vi "Grab Image.vi"(8 "error in (no error)":errorcluster, 11 "Bobcat 640 in":refnum<class "Bobcat 640.lvclass">) -> (0 "error out":errorcluster, 3 "Bobcat 640 out":refnum<class "Bobcat 640.lvclass">)   [LabVIEW 2018, in "Bobcat 640.lvlib" / "Bobcat 640.lvclass"]
uses:
  Bobcat 640.lvclass
  Bobcat 640.lvclass/Bobcat 640.ctl
  PPLs/Camera/Parent/Camera.lvlibp/Camera.lvclass
  <vilib>/vision/driver/NI_Vision_Acquisition_Software.lvlib
  C:/AME Test Engineering/LabVIEW/PPLs/Camera/Parent/Camera.lvlibp/Camera.lvclass
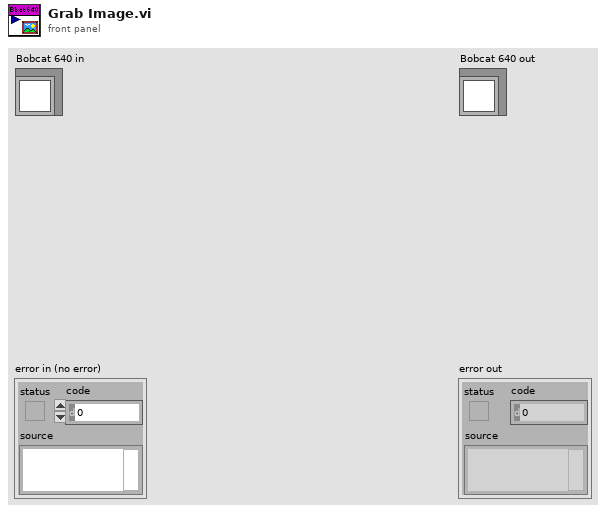
[diagram p1: front panel]
types:
  T1 = typedef "IMAQdx.ctl" = refnum<k21>
  T2 = typedef "Camera.lvlibp/IMAQ Image.ctl" = refnum<image>
  T3 = typedef "IMAQ Image.ctl" = refnum<image>
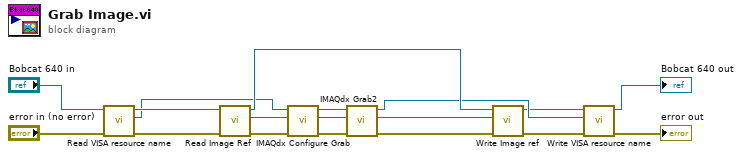
[diagram p0: block diagram]
diagram:
  n1 = call "Read VISA resource name.vi"("error in (no error)"="error in (no error)", "Bobcat 640 in"="Bobcat 640 in") -> ("error out"=w5:errorcluster, "IMAQdx Session"=w4:T1, "Bobcat 640 out"=w6:refnum<class "Bobcat 640.lvclass">)  [unwired: 7 in]
  n2 = call "Read Image Ref.vi"("error in (no error)"=w5, "Camera in"=w6) -> ("error out"=w3:errorcluster, "Image"=w7:T2, "Camera out"=w12:refnum<class "Bobcat 640.lvclass">)  [unwired: 7 in]
  n3 = call <vilib>:"IMAQdx Configure Grab.vi"("error in"=w3, "Session In"=w4) -> ("error out"=w1:errorcluster, "Session Out"=w2:T1)  [unwired: 8 in]
  n4 = call <vilib>:"IMAQdx Grab2.vi"("error in"=w1, "Image In"=w7, "Session In"=w2) -> ("error out"=w11:errorcluster, "Image Out"=w13:T3, "Session Out"=w10:T1)  [unwired: 5 in, 1 out]
  n5 = call "Write Image ref.vi"("error in (no error)"=w11, "Image"=w13, "Camera in"=w12) -> ("error out"=w8:errorcluster, "Camera out"=w9:refnum<class "Bobcat 640.lvclass">)  [unwired: 7 in]
  n6 = call "Write VISA resource name.vi"("error in (no error)"=w8, "IMAQdx Session"=w10, "Bobcat 640 in"=w9) -> ("error out"=→"error out":errorcluster, "Bobcat 640 out"=→"Bobcat 640 out":refnum<class "Bobcat 640.lvclass">)  [unwired: 7 in]
